vi "WLAN_SuperposedFrameBuild.vi"(7 "Alpha":dbl min=0.0 max=1.0 step=0.05 format="%#_13g", 8 "error in (no error)":errorcluster, 9 "data in 2":i8[](array[numeric]) caption="input bit stream", 10 "Modulation parameter":T1, 11 "data in":i8[](array[numeric]) caption="input bit stream") -> (0 "error out":errorcluster, 3 "output array":cdb[](array[numeric]))   [LabVIEW 2022 SP3]
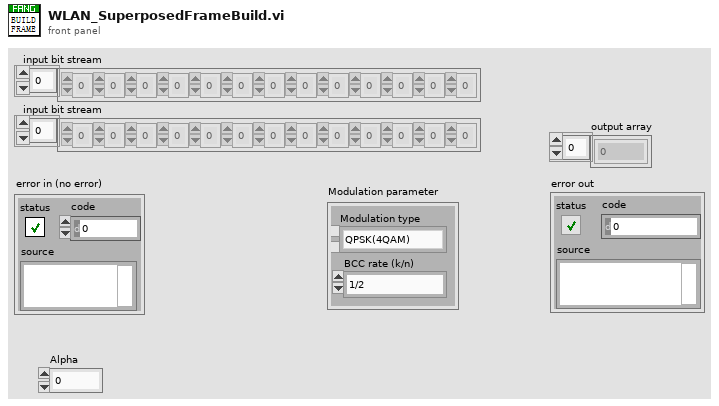
[diagram p1: front panel]
types:
  T1 = cluster{"Modulation type":enum16{"QPSK(4QAM)", "64QAM", "16QAM", "BPSK"}, "BCC rate (k/n)":enum16{"1/2", "2/3", "3/4"}}
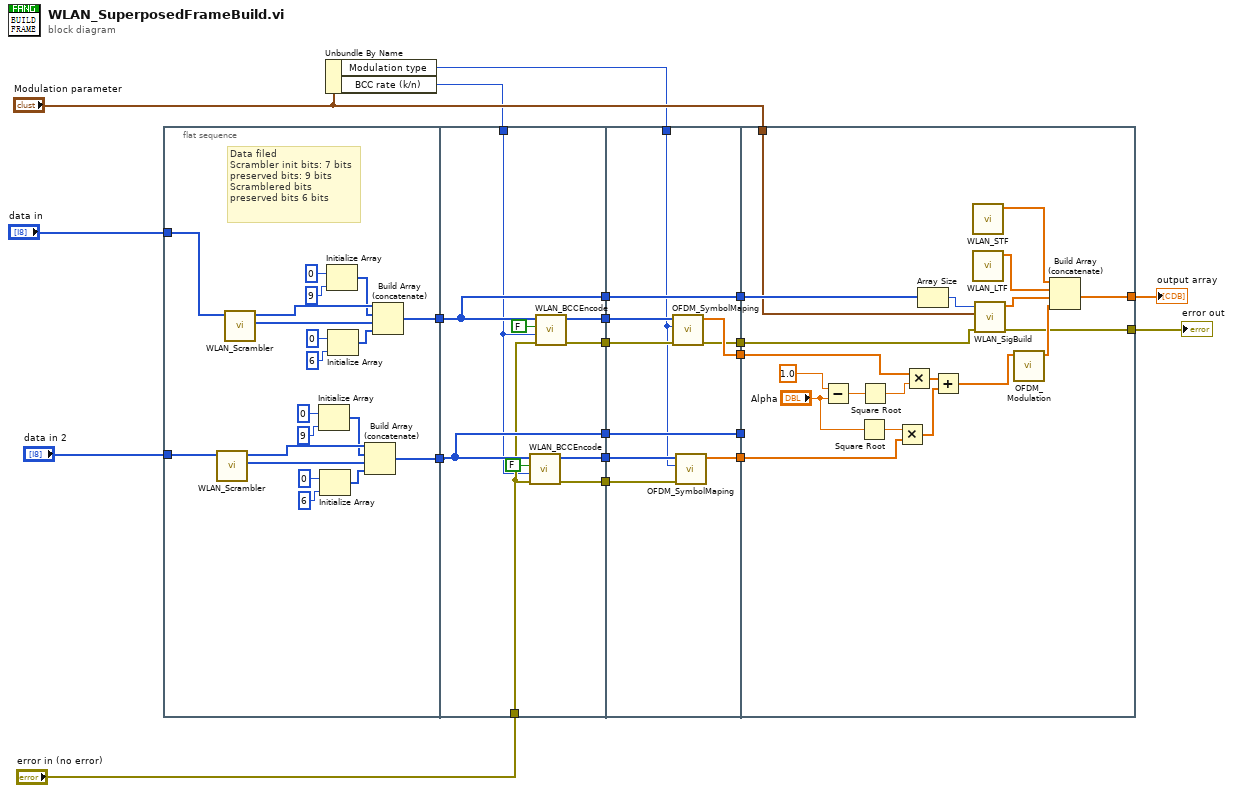
[diagram p0: block diagram]
diagram:
  n1 = flat-sequence {
    tunnel: "data in" -> [w33]
    tunnel: [w32] -> w20
    tunnel: "data in 2" -> [w23]
    tunnel: [w22] -> w6
    tunnel: w20 -> [w48]
    tunnel: "error in (no error)" -> [w44]
    tunnel: [w50] -> w18
    tunnel: [w49] -> w17
    tunnel: w14 -> [w43]
    tunnel: [w48] -> w9
    tunnel: w6 -> [w46]
    tunnel: [w46] -> w5
    tunnel: [w45] -> w4
    tunnel: [w42] -> w2
    tunnel: w18 -> [w61]
    tunnel: w17 -> [w60]
    tunnel: w15 -> [w54]
    tunnel: [w59] -> w13
    tunnel: [w58] -> w12
    tunnel: w9 -> [w57]
    tunnel: [w57] -> w8
    tunnel: w5 -> [w55]
    tunnel: w4 -> [w56]
    tunnel: [w55] -> w3
    tunnel: w2 -> [w53]
    tunnel: [w52] -> w1
    tunnel: "Modulation parameter" -> [w79]
    tunnel: w13 -> [w64]
    tunnel: w12 -> [w74]
    tunnel: [w73] -> w11
    tunnel: [w72] -> w10
    tunnel: w8 -> [w81]
    tunnel: w3 -> [_]
    tunnel: w1 -> [w63]
    frame #0 {
      # "Data filed\nScrambler init bits: 7 bits\npreserved bits: 9 bits\nScramblered bits\npreserved bits 6 bits"
      n2 = call "WLAN_Scrambler.vi"("input bit stream"=w23) -> ("scrambled bits"=w27:i8[], "scrambler initial bit"=w31:i8[])  [unwired: 9 in]
      n3 = call "WLAN_Scrambler.vi"("input bit stream"=w33) -> ("scrambled bits"=w37:i8[], "scrambler initial bit"=w41:i8[])  [unwired: 9 in]
      n4 = Initialize Array(i8 0 ("element"), 9 ("dimension size")) -> (w30:i8[])
      n5 = Initialize Array(i8 0 ("element"), 6 ("dimension size")) -> (w24:i8[])
      n6 = Initialize Array(i8 0 ("element"), 9 ("dimension size")) -> (w40:i8[])
      n7 = Initialize Array(i8 0 ("element"), 6 ("dimension size")) -> (w34:i8[])
      n8 = Build Array (concatenate)(w31, w30, w27, w24) -> (w22:i8[])
      n9 = Build Array (concatenate)(w41, w40, w37, w34) -> (w32:i8[])
    }
    frame #1 {
      n10 = call "WLAN_BCCEncode.vi"("error in (no error)"=w44, "BCC rate (k/n)"=w43, "need add zeros?"=FALSE, "input bit stream"=w46) -> ("error out"=w42:errorcluster, "output bit stream 3"=w45:i8[])  [unwired: 6 in]
      n11 = call "WLAN_BCCEncode.vi"("error in (no error)"=w44, "BCC rate (k/n)"=w43, "need add zeros?"=FALSE, "input bit stream"=w48) -> ("error out"=w50:errorcluster, "output bit stream 3"=w49:i8[])  [unwired: 6 in]
    }
    frame #2 {
      n12 = call "OFDM_SymbolMaping.vi"("error in (no error)"=w61, "Modulation type"=w54, "input bit stream"=w60) -> ("error out"=w58:errorcluster, "symbols"=w59:cdb[])  [unwired: 7 in]
      n13 = call "OFDM_SymbolMaping.vi"("error in (no error)"=w53, "Modulation type"=w54, "input bit stream"=w56) -> ("symbols"=w52:cdb[])  [unwired: 7 in, 1 out]
    }
    frame #3 {
      n14 = Subtract(x=1.0, y="Alpha") -> (x-y=w66:dbl)
      n15 = Square Root(x="Alpha") -> (sqrt(x)=w70:dbl)
      n16 = Square Root(x=w66) -> (sqrt(x)=w68:dbl)
      n17 = Multiply(x=w70, y=w63) -> (x*y=w71:cdb[])
      n18 = Multiply(x=w64, y=w68) -> (x*y=w69:cdb[])
      n19 = Array Size(array=w81) -> (size(s)=w80:i32)
      n20 = Add(x=w69, y=w71) -> (x+y=w62:cdb[])
      n21 = call "WLAN_STF.vi"() -> ("STF"=w75:cdb[])  [unwired: 11 in]
      n22 = call "WLAN_LTF.vi"() -> ("LTF"=w76:cdb[])  [unwired: 11 in]
      n23 = call "WLAN_SigBuild.vi"("Data bit length"=w80, "Modulation parameter"=w79, "error in (no error)"=w74) -> ("symbols"=w77:cdb[], "error out"=w73:errorcluster)  [unwired: 6 in]
      n24 = call "OFDM_Modulation.vi"("Input sequence"=w62) -> ("Output sequence"=w78:cdb[])  [unwired: 10 in]
      n25 = Build Array (concatenate)(w75, w76, w77, w78) -> (w72:cdb[])
    }
  }
  n26 = Unbundle By Name("Modulation parameter") -> ("Modulation type"=w15:enum16{"QPSK(4QAM)", "64QAM", "16QAM", "BPSK"}, "BCC rate (k/n)"=w14:enum16{"1/2", "2/3", "3/4"})
  "output array" <- w10
  "error out" <- w11
